vi "Main.vi"() -> ()   [LabVIEW 2014]
uses:
  <vilib>/Utility/sysdir.llb/System Directory Type.ctl
panel:
  out "Application:Kind":T1(ring)
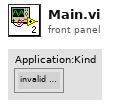
[diagram p1: front panel]
types:
  T1 = enum32{"invalid app kind", "Development System", "Run Time System", "Student Edition", "Embedded LabVIEW", "Evaluation", "Custom"}
  T2 = typedef "System Directory Type.ctl" = i32
  T3 = cluster{"Position of Robot":string, "Comments":string, "Did Your Robot Move a Can\n into Auto Zone":string, "Did Your Robot Move a Crate\n into Auto Zone ":string, "Is Your Robot in Auto Zone":string, "Team Number":string}
  T4 = enum16{"open", "replace", "create", "open or create", "replace or create", "replace or create with confirmation"}
  T5 = cluster{"Comments":string, dbl, dbl, dbl, dbl, dbl, dbl, dbl, dbl, dbl, "Can They Move Litter to Landfill":string}
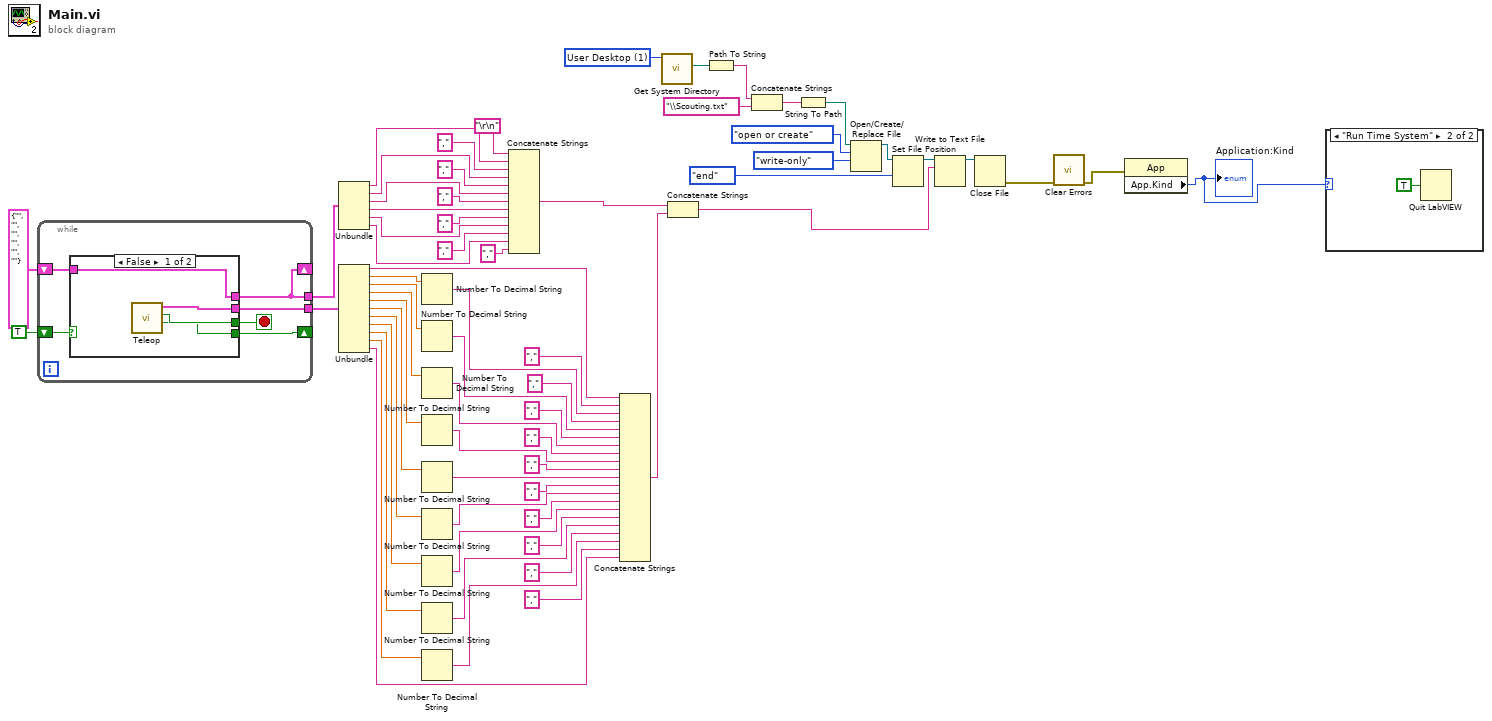
[diagram p0: block diagram]
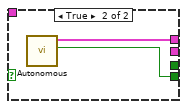
[diagram p3: hidden frame]
diagram:
  w9 = T2 1 items=["User Home"=0, "User Desktop"=1, "User Documents"=2, "User Application Data"=3, "User Preferences"=4, "User Temporary"=5, "Public Documents"=6, "Public Application Data"=7, "Public Preferences"=8, "Public Cache"=13, "System Core Libraries"=9, "System Installed Libraries"=10, "Application Files"=11, "Boot Volume Root"=12] ("system directory type")
  n1 = while {
    shift-right: [w71] -> _
    shift-left: TRUE ("Boolean") -> [w70]
    tunnel: [w67] -> w60
    tunnel: [w68] -> w61
    shift-right: [w67] -> _
    shift-left: T3 {"Position of Robot"="", "Comments"="", "Did Your Robot Move a Can\n into Auto Zone"="", "Did Your Robot Move a Crate\n into Auto Zone "="", "Is Your Robot in Auto Zone"="", "Team Number"=""} ("output cluster") -> [w66]
    stop <- w69 stop-if-true
    n2 = case shown="False" w70 {
      tunnel: [w72 w77] -> w71
      tunnel: [w74 w76] -> w67
      tunnel: [w73 _] -> w69
      tunnel: [w75 _] -> w68
      tunnel: w66 -> [w74 _]
      frame False {
        n3 = call "Teleop.vi"() -> ("Boolean"=w72:bool, "Boolean 2"=w73:bool, "output cluster"=w75:T5)  [unwired: 8 in]
      }
      frame True {
        n4 = call "Autonomous.vi"() -> ("Boolean"=w77:bool, "output cluster"=w76:T3)  [unwired: 10 in]
      }
    }
  }
  n5 = Unbundle(w60) -> ("Position of Robot"=w57:string, "Comments"=w56:string, "Did Your Robot Move a Can\n into Auto Zone"=w55:string, "Did Your Robot Move a Crate\n into Auto Zone"=w54:string, "Is Your Robot in Auto Zone"=w53:string, "Team Number"=w52:string)
  n6 = Unbundle(w61) -> ("Comments"=w59:string, w35:dbl, w33:dbl, w31:dbl, w29:dbl, w27:dbl, w25:dbl, w23:dbl, w21:dbl, w18:dbl, "Can They Move Litter to Landfill"=w58:string)
  n7 = Number To Decimal String(number=w35) -> (decimal integer string=w34:string)  [unwired: 1 in]
  n8 = Number To Decimal String(number=w33) -> (decimal integer string=w32:string)  [unwired: 1 in]
  n9 = Number To Decimal String(number=w31) -> (decimal integer string=w30:string)  [unwired: 1 in]
  n10 = Number To Decimal String(number=w29) -> (decimal integer string=w28:string)  [unwired: 1 in]
  n11 = Number To Decimal String(number=w27) -> (decimal integer string=w26:string)  [unwired: 1 in]
  n12 = Number To Decimal String(number=w25) -> (decimal integer string=w24:string)  [unwired: 1 in]
  n13 = Number To Decimal String(number=w23) -> (decimal integer string=w22:string)  [unwired: 1 in]
  n14 = Number To Decimal String(number=w21) -> (decimal integer string=w20:string)  [unwired: 1 in]
  n15 = Number To Decimal String(number=w18) -> (decimal integer string=w19:string)  [unwired: 1 in]
  n16 = Concatenate Strings("\r\n", w57, ",", w56, ",", w55, ",", w54, ",", w53, ",", w52, ",") -> (w16:string)
  n17 = Concatenate Strings(w59, ",", w34, ",", w32, ",", w30, ",", w28, ",", w26, ",", w24, ",", w22, ",", w20, ",", w19, ",", w58) -> (w17:string)
  n18 = call <vilib>:"Get System Directory.vi"("system directory type"=w9) -> ("system directory"=w8:path)  [unwired: 10 in]
  n19 = Concatenate Strings(w16, w17) -> (w15:string)
  n20 = Path To String(path=w8) -> (string=w7:string)
  n21 = Concatenate Strings(w7, "\\Scouting.txt" ("string")) -> (w5:string)
  n22 = String To Path(string=w5) -> (path=w4:path)
  n23 = Open/Create/Replace File(file path (use dialog)=w4, operation (0:open)=T4."open or create", access (0:read/write)=enum16{"read/write", "read-only", "write-only"}."write-only") -> (refnum out=w12:refnum<file>)  [unwired: 3 in, 2 out]
  n24 = Set File Position(refnum=w12, from (0:start)=enum16{"start", "end", "current"}."end") -> (refnum out=w11:refnum<file>)  [unwired: 2 in, 1 out]
  n25 = Write to Text File(file (use dialog)=w11, text=w15) -> (refnum out=w62:refnum<file>)  [unwired: 2 in, 2 out]
  n26 = Close File(refnum=w62) -> (error out=w3:errorcluster)  [unwired: 1 in, 1 out]
  n27 = call <vilib>:"Clear Errors.vi"("error in (no error)"=w3) -> ("error out"=w2:errorcluster)  [unwired: 5 in, 1 out]
  n28 = property class="App"(error in=w2) -> ("App.Kind"=w1:T1)  [unwired: 1 in, 2 out]
  "Application:Kind" <- w1
  n29 = case shown="\"Run Time System\"" w1 {
    frame Default {
    }
    frame "Run Time System" {
      n30 = Quit LabVIEW(quit? (T)=TRUE) -> ()
    }
  }
